vi "Find Position.vi"(8 "error in (no error)":errorcluster, 11 "Circular Buffer in":refnum<class "Circular Buffer.lvclass">) -> (0 "error out":errorcluster, 2 "Position":i32, 3 "Circular Buffer out":refnum<class "Circular Buffer.lvclass">)   [LabVIEW 2021]
uses:
  Node.ctl
  Circular Buffer.lvclass
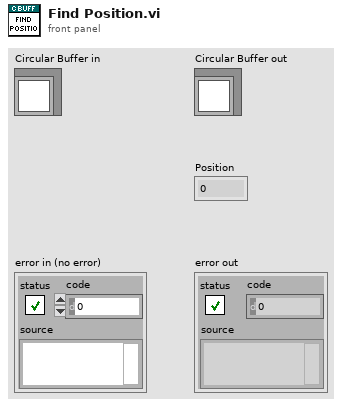
[diagram p1: front panel]
types:
  T1 = typedef "d20.lvlib/Circular Buffer.lvclass/Node.ctl" = cluster{"Shift":i32, "previous":refnum<data-value>, "next":refnum<data-value>, "Decription":i64}
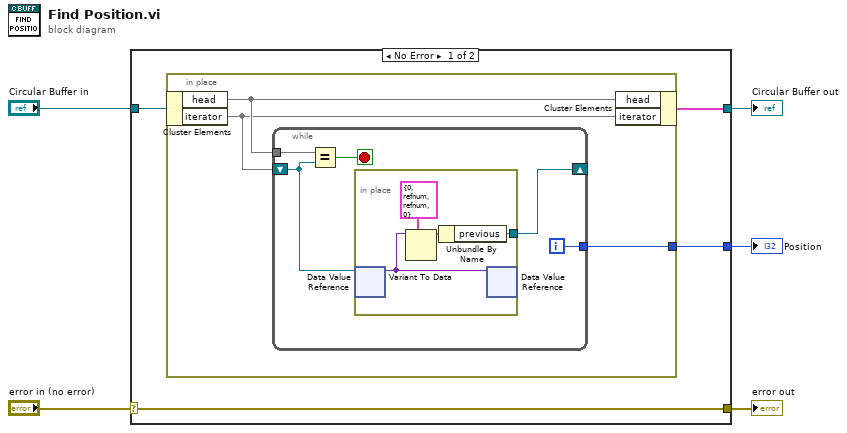
[diagram p0: block diagram]
diagram:
  n1 = case shown="No Error" "error in (no error)" {
    selector: "error in (no error)" -> [w9 w23]
    tunnel: [w9 w23] -> w4
    tunnel: [w6 w22] -> w2
    tunnel: "Circular Buffer in" -> [w7 w22]
    tunnel: [w8 _] -> w1
    frame No Error {
      n2 = in-place {
        in-place-border: [w12] -> w8
        n3 = in-place-cluster #1(w7) -> ("head"=w11, "iterator"=w10)
        n4 = while {
          shift-right: [w14] -> _
          shift-left: w10 -> [w15]
          tunnel: [w16] -> w12
          tunnel: w11 -> [w13]
          i -> [w16]
          stop <- w17 stop-if-true
          n5 = Equal?(x=w13, y=w15) -> (x = y?=w17:bool)
          n6 = in-place {
            in-place-border: [w18] -> w14
            n7 = in-place-dvr #2(w15) -> (w21:variant)  [unwired: 1 out]
            n8 = Variant To Data(type=T1 {"Shift"=0, "previous"=refnum, "next"=refnum, "Decription"=0} ("Doubly Linked List"), Variant=w21) -> (data=w19:T1)  [unwired: 1 in, 1 out]
            n9 = Unbundle By Name(w19) -> ("previous"=w18:refnum<data-value>)
            n10 = in-place-dvr #2(w21) -> ()  [unwired: 2 out]
          }
        }
        n11 = in-place-cluster #1("head"=w11, "iterator"=w10) -> (w6:cluster{})
      }
    }
    frame Error {
    }
  }
  "error out" <- w4
  "Circular Buffer out" <- w2
  "Position" <- w1
